vi "Heapify.vi"(1 "Index":i32, 2 "Length":i32, 3 "Array":T1[](array[typedef])) -> (0 "Heapified Array":T1[](array[typedef]))   [LabVIEW 2018]
uses:
  Graham Scan Point.ctl
  d7b2d06d-9c24-460d-8352-84b3877a1686.vi
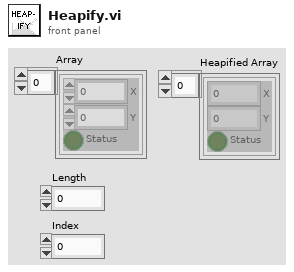
[diagram p1: front panel]
types:
  T1 = typedef "Graham Scan Point.ctl" = cluster{"X":i32, "Y":i32, "Status":bool}
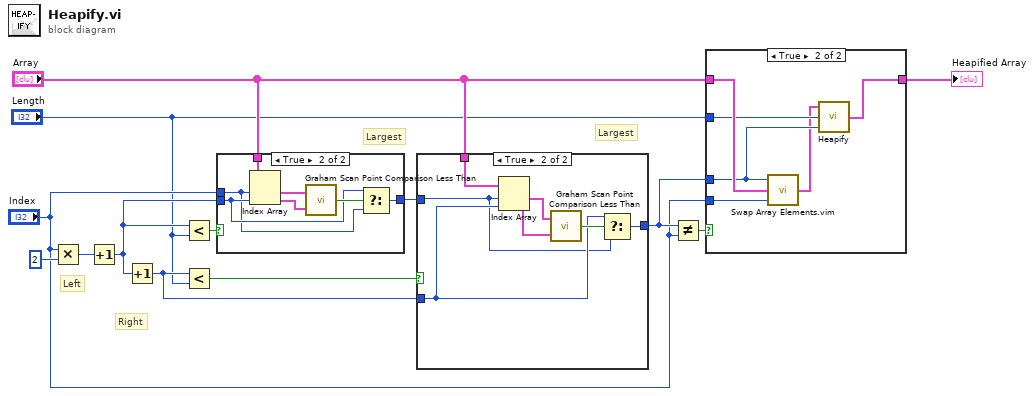
[diagram p0: block diagram]
diagram:
  # "Largest"
  # "Largest"
  # "Right"
  # "Left"
  n1 = Multiply(x="Index", y=2) -> (x*y=w12:i32)
  n2 = Increment(x=w12) -> (x+1=w10:i32)
  n3 = Increment(x=w10) -> (x+1=w7:i32)
  n4 = Less?(x=w10, y="Length") -> (x < y?=w11:bool)
  n5 = Less?(x=w7, y="Length") -> (x < y?=w9:bool)
  n6 = case shown="True" w11 {
    tunnel: "Array" -> [_ w21]
    tunnel: w10 -> [_ w17]
    tunnel: "Index" -> [w14 w16]
    tunnel: [w14 w15] -> w8
    frame False {
    }
    frame True {
      n7 = Index Array(array=w21, index #1=w16, index #2=w17) -> (element #1=w20:T1, element #2=w19:T1)
      n8 = call "Graham Scan Point Comparison Less Than.vi"("B"=w19, "A"=w20) -> ("A < B?"=w18:bool)
      n9 = Select(t=w17, s=w18, f=w16) -> (s? t:f=w15:i32)
    }
  }
  n10 = case shown="True" w9 {
    tunnel: w8 -> [w22 w24]
    tunnel: w7 -> [_ w25]
    tunnel: "Array" -> [_ w29]
    tunnel: [w22 w23] -> w4
    frame False {
    }
    frame True {
      n11 = Index Array(array=w29, index #1=w24, index #2=w25) -> (element #1=w28:T1, element #2=w27:T1)
      n12 = call "Graham Scan Point Comparison Less Than.vi"("B"=w27, "A"=w28) -> ("A < B?"=w26:bool)
      n13 = Select(t=w25, s=w26, f=w24) -> (s? t:f=w23:i32)
    }
  }
  n14 = Not Equal?(x=w4, y="Index") -> (x != y?=w6:bool)
  n15 = case shown="True" w6 {
    tunnel: "Array" -> [w30 w35]
    tunnel: w4 -> [_ w33]
    tunnel: "Index" -> [_ w36]
    tunnel: "Length" -> [_ w34]
    tunnel: [w30 w31] -> w1
    frame False {
    }
    frame True {
      n16 = call "Swap Array Elements.vim"("Index B"=w36, "Array"=w35, "Index A"=w33) -> ("Array Out"=w32:T1[])
      n17 = call "Heapify.vi"("Index"=w33, "Length"=w34, "Array"=w32) -> ("Heapified Array"=w31:T1[])
    }
  }
  "Heapified Array" <- w1
